vi "WW_GatherSpinParameter.vi"(2 "路径":path) -> (0 "ProgressFinalSpin":T4, 1 "FinalSpinEnd_Index":u32, 3 "RUNStateID":T1, 4 "EXCEL读取":string[][](array[string]), 5 "ProgressInitial":T3, 6 "POWERStateID":T2)   [LabVIEW 2011]
panel:
  # "常用参数：\nPogress_FinalSpin_Index:  用于存储PogressFinalSpinIndex, 用于标定\nFinalSpin_SetpDrain: 用于存储SepDain, 标定\nFinalSpin_StepSpin: 用于活动Spin阶段，进行时间比较\nFinalSpin_StepLoose: 用于活动Loose阶段，标定，而后开始比较"
  # "常用参数：\nPOWER_UPSTGART_Index： 整机正在上电\nPOWER_ON_Idex： 整机处于完全上电状态"
  # "常用参数：\nInitial_StepFirstDrain,(用于计算差价)"
  # "常用参数：\nRUNMODE_READY_Index : 整机准备运行状态\nRUNMODE_RUNNING_Index : 整机处于运行状态"
  # "常用参数：\nFinalSpinEnd_Index: 用于表示数据比对结束"
  # "Useful"
  # "Useful"
  # "Useful"
  # "Useful"
  # "Useful"
  # "Useful"
  # "Useful"
  # "Useful"
  # "Useful"
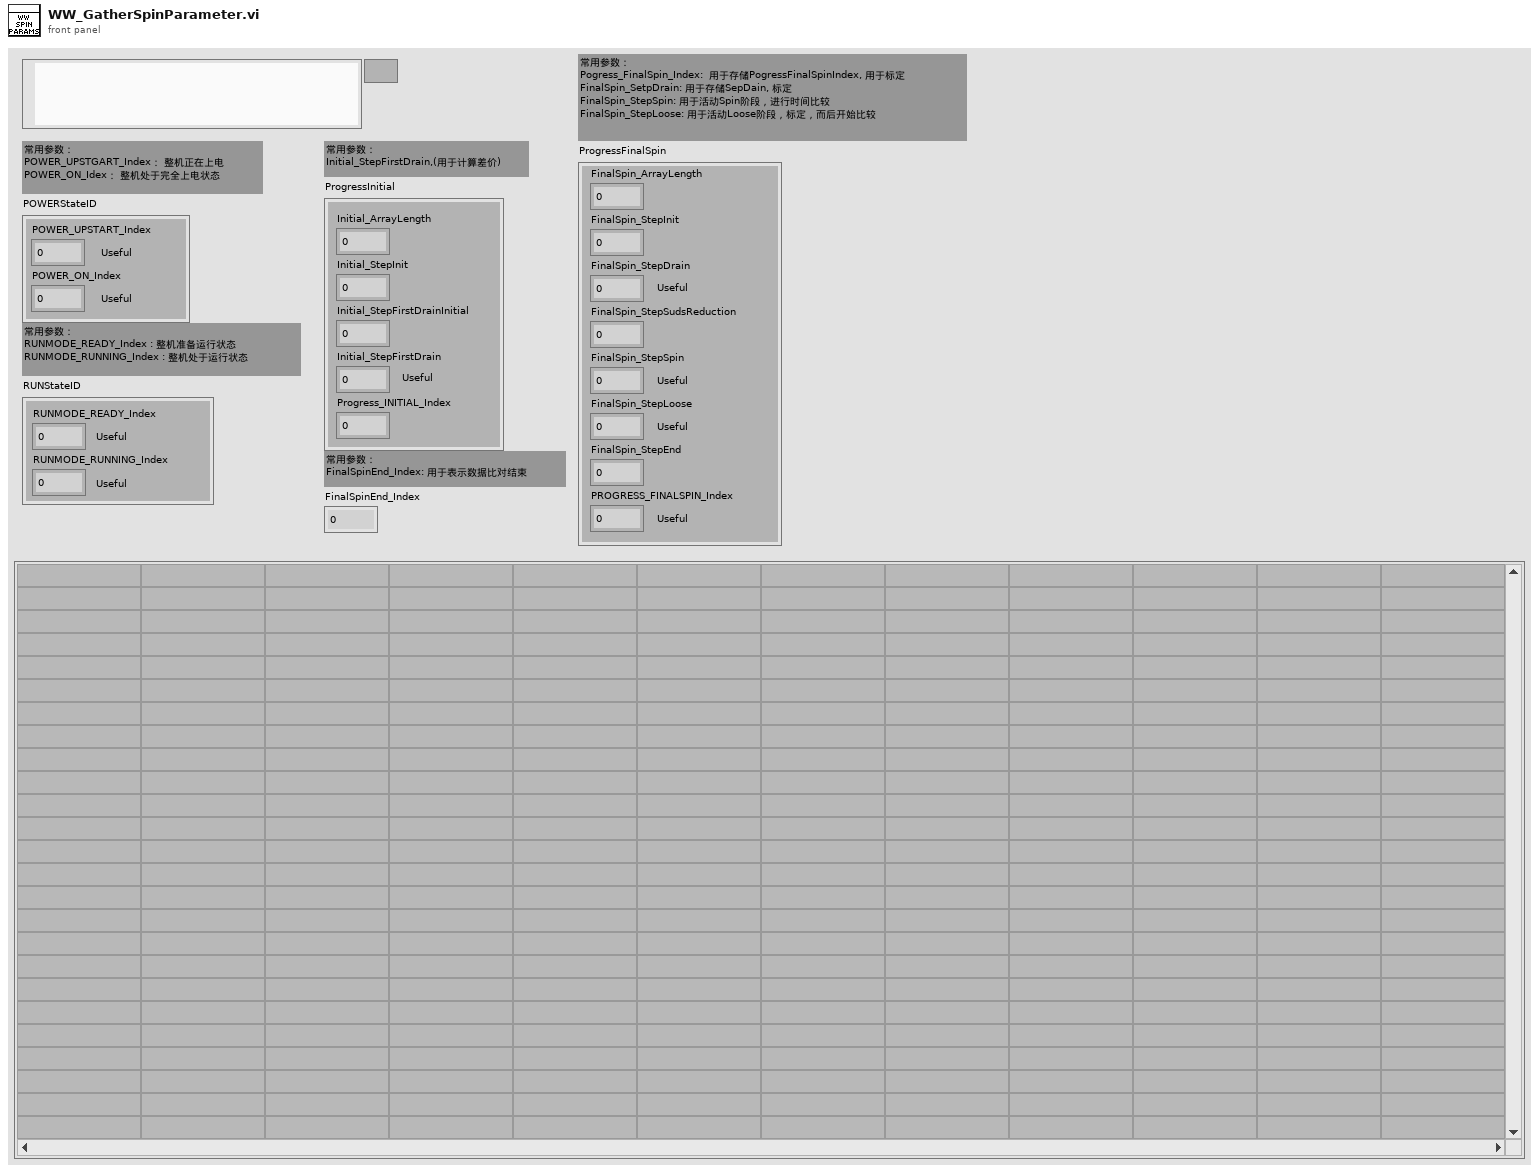
[diagram p1: front panel]
types:
  T1 = cluster{"RUNMODE_READY_Index":u32, "RUNMODE_RUNNING_Index":u32}
  T2 = cluster{"POWER_UPSTART_Index":u32, "POWER_ON_Index":u32}
  T3 = cluster{"Initial_ArrayLength":u32, "Initial_StepInit":u32, "Initial_StepFirstDrainInitial":u32, "Initial_StepFirstDrain":u32, "Progress_INITIAL_Index":u32}
  T4 = cluster{"FinalSpin_ArrayLength":u32, "FinalSpin_StepInit":u32, "FinalSpin_StepDrain":u32, "FinalSpin_StepSudsReduction":u32, "FinalSpin_StepSpin":u32, "FinalSpin_StepLoose":u32, "FinalSpin_StepEnd":u32, "PROGRESS_FINALSPIN_Index":u32}
  T5 = enum16{"RealTime", "WaterLevel", "WaterTemp", "AirTemp", "IPMTemp", "MotorActualRPM", "MotorTargetRPM", "FanActualRPM", "MemsSensorA", "MemsSensorB", "MemsSensorC", "WaterThermistorADC", "TouchSensor", "LeakageSensor", "DCLink", "IsDoorOpen", "IsTimeShort", "Progress", "Step", "TotalRemainTime", "StepRemainTime", "WeightSensingLowData", "WeightSensingResult", "ColdValve", "HotValve", "PreValve", "WaterShotValve", "BleachValve", "DryValve", "SteamValve", "SoftenerValve", "FilterValve", "IsDoorLocked", "SSRCommon", "MainRelay", "ACTUATOR2", "WaterDrainer", "CirculationPump", "WaterHeater", "DryHeater", "SteamHeater", "MotorDriveDirection", "IsDoubleDoorOpen", "IsDoubleDoorLock", "RunStateID", "PowerStateID", "SoundID", "ErrorCode", "OptionData", "MainVersion", "SUBVersion", "InverterVersion"}
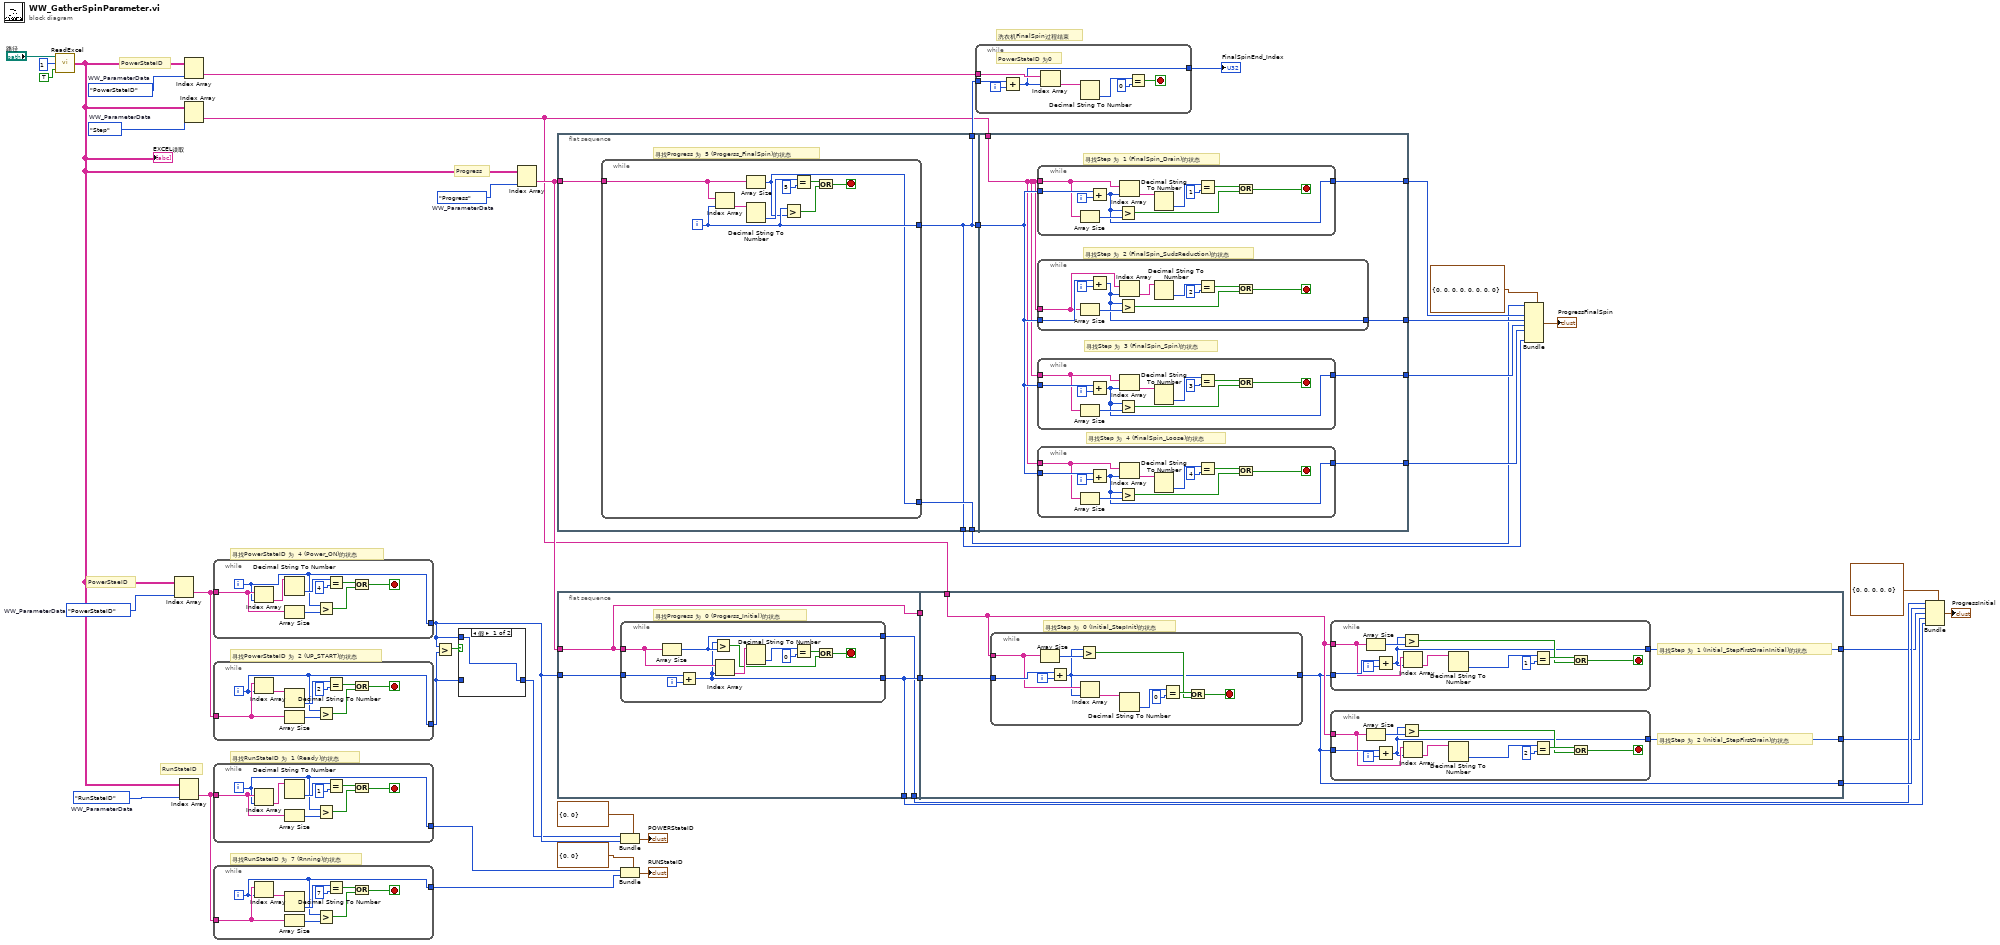
[diagram p0: block diagram]
diagram:
  w6 = T5."RunStateID"  # WW_ParameterData
  w7 = T5."PowerStateID"  # WW_ParameterData
  w9 = T5."Step"  # WW_ParameterData
  w10 = T5."Progress"  # WW_ParameterData
  w11 = T5."PowerStateID"  # WW_ParameterData
  # "PowerStaeID"
  # "洗衣机FinalSpin过程结束"
  # "Progress"
  # "PowerStateID"
  # "RunStateID"
  # "寻找PowerStateID 为  4 (Power_ON)的状态"
  # "寻找PowerStateID 为  2 (UP_START)的状态"
  # "寻找RunStateID 为  1 (Ready)的状态"
  # "寻找RunStateID 为  7 (Rnning)的状态"
  n1 = call "ReadExcel.vi"("读出文本"=TRUE, "导出sheet位号"=i8 1, "路径"="路径") -> ("EXCEL读取"=w12:string[][])
  "EXCEL读取" <- w12
  n2 = Index Array(array=w12, index (col)=w7) -> (element=w40:string[])  [unwired: 1 in]
  n3 = Index Array(array=w12, index (col)=w6) -> (element=w41:string[])  [unwired: 1 in]
  n4 = Index Array(array=w12, index (col)=w11) -> (element=w20:string[])  [unwired: 1 in]
  n5 = Index Array(array=w12, index (col)=w9) -> (element=w8:string[])  [unwired: 1 in]
  n6 = while {
    tunnel: w40 -> [w51]
    tunnel: [w49] -> w2
    i -> [w49]
    stop <- w45 stop-if-true
    n7 = Index Array(array=w51, index=w49) -> (element=w53:string)
    n8 = Decimal String To Number(string=w53) -> (number=w52:i32)  [unwired: 2 in, 1 out]
    n9 = Array Size(array=w51) -> (size(s)=w48:i32)
    n10 = Greater?(x=w49, y=w48) -> (0:w46:bool)
    n11 = Equal?(x=w52, y=4) -> (x = y?=w47:bool)
    n12 = Or(x=w47, y=w46) -> (x .or. y?=w45:bool)
  }
  n13 = while {
    tunnel: w40 -> [w60]
    tunnel: [w58] -> w3
    i -> [w58]
    stop <- w54 stop-if-true
    n14 = Index Array(array=w60, index=w58) -> (element=w62:string)
    n15 = Decimal String To Number(string=w62) -> (number=w61:i32)  [unwired: 2 in, 1 out]
    n16 = Array Size(array=w60) -> (size(s)=w57:i32)
    n17 = Greater?(x=w58, y=w57) -> (0:w55:bool)
    n18 = Equal?(x=w61, y=2) -> (x = y?=w56:bool)
    n19 = Or(x=w56, y=w55) -> (x .or. y?=w54:bool)
  }
  n20 = while {
    tunnel: w41 -> [w69]
    tunnel: [w67] -> w14
    i -> [w67]
    stop <- w63 stop-if-true
    n21 = Index Array(array=w69, index=w67) -> (element=w71:string)
    n22 = Decimal String To Number(string=w71) -> (number=w70:i32)  [unwired: 2 in, 1 out]
    n23 = Array Size(array=w69) -> (size(s)=w66:i32)
    n24 = Greater?(x=w67, y=w66) -> (0:w64:bool)
    n25 = Equal?(x=w70, y=1) -> (x = y?=w65:bool)
    n26 = Or(x=w65, y=w64) -> (x .or. y?=w63:bool)
  }
  n27 = while {
    tunnel: w41 -> [w78]
    tunnel: [w76] -> w13
    i -> [w76]
    stop <- w72 stop-if-true
    n28 = Index Array(array=w78, index=w76) -> (element=w80:string)
    n29 = Decimal String To Number(string=w80) -> (number=w79:i32)  [unwired: 2 in, 1 out]
    n30 = Array Size(array=w78) -> (size(s)=w75:i32)
    n31 = Greater?(x=w76, y=w75) -> (0:w73:bool)
    n32 = Equal?(x=w79, y=7) -> (x = y?=w74:bool)
    n33 = Or(x=w74, y=w73) -> (x .or. y?=w72:bool)
  }
  n34 = Greater?(x=w2, y=w3) -> (0:w5:bool)
  n35 = case shown="假" w5 {
    tunnel: w3 -> [_ w82]
    tunnel: w2 -> [w81 _]
    tunnel: [w81 w82] -> w1
    frame False {
    }
    frame True {
    }
  }
  n36 = Index Array(array=w12, index (col)=w10) -> (element=w28:string[])  [unwired: 1 in]
  n37 = flat-sequence {
    tunnel: w28 -> [w85]
    tunnel: [w83] -> w39
    tunnel: [w83] -> w32
    tunnel: [w84] -> w31
    tunnel: [w83] -> w19
    tunnel: w39 -> [w97]
    tunnel: w8 -> [w96]
    tunnel: [w100] -> w37
    tunnel: [w99] -> w36
    tunnel: [w98] -> w35
    tunnel: [w95] -> w34
    frame #0 {
      # "寻找Progress 为  5 (Progerss_FinalSpin)的状态"
      n38 = while {
        tunnel: w85 -> [w91]
        tunnel: [w87] -> w83
        tunnel: [w86] -> w84
        i -> [w87]
        stop <- w88 stop-if-true
        n39 = Index Array(array=w91, index=w87) -> (element=w94:string)
        n40 = Array Size(array=w91) -> (size(s)=w86:i32)
        n41 = Decimal String To Number(string=w94) -> (number=w93:i32)  [unwired: 2 in, 1 out]
        n42 = Greater?(x=w87, y=w86) -> (0:w89:bool)
        n43 = Equal?(x=w93, y=5) -> (x = y?=w90:bool)
        n44 = Or(x=w90, y=w89) -> (x .or. y?=w88:bool)
      }
    }
    frame #1 {
      # "寻找Step 为  4 (FinalSpin_Loose)的状态"
      # "寻找Step 为  3 (FinalSpin_Spin)的状态"
      # "寻找Step 为  2 (FinalSpin_SudsReduction)的状态"
      # "寻找Step 为  1 (FinalSpin_Drain)的状态"
      n45 = while {
        tunnel: w97 -> [w144]
        tunnel: w96 -> [w134]
        tunnel: [w135] -> w100
        i -> [w143]
        stop <- w136 stop-if-true
        n46 = Array Size(array=w134) -> (size(s)=w139:i32)
        n47 = Add(x=w144, y=w143) -> (x+y=w135:i32)
        n48 = Greater?(x=w135, y=w139) -> (0:w137:bool)
        n49 = Index Array(array=w134, index=w135) -> (element=w142:string)
        n50 = Decimal String To Number(string=w142) -> (number=w141:i32)  [unwired: 2 in, 1 out]
        n51 = Equal?(x=w141, y=1) -> (x = y?=w138:bool)
        n52 = Or(x=w138, y=w137) -> (x .or. y?=w136:bool)
      }
      n53 = while {
        tunnel: w97 -> [w133]
        tunnel: w96 -> [w123]
        tunnel: [w124] -> w99
        i -> [w132]
        stop <- w125 stop-if-true
        n54 = Array Size(array=w123) -> (size(s)=w128:i32)
        n55 = Add(x=w133, y=w132) -> (x+y=w124:i32)
        n56 = Greater?(x=w124, y=w128) -> (0:w126:bool)
        n57 = Index Array(array=w123, index=w124) -> (element=w131:string)
        n58 = Decimal String To Number(string=w131) -> (number=w130:i32)  [unwired: 2 in, 1 out]
        n59 = Equal?(x=w130, y=2) -> (x = y?=w127:bool)
        n60 = Or(x=w127, y=w126) -> (x .or. y?=w125:bool)
      }
      n61 = while {
        tunnel: w97 -> [w122]
        tunnel: w96 -> [w112]
        tunnel: [w113] -> w98
        i -> [w121]
        stop <- w114 stop-if-true
        n62 = Array Size(array=w112) -> (size(s)=w117:i32)
        n63 = Add(x=w122, y=w121) -> (x+y=w113:i32)
        n64 = Greater?(x=w113, y=w117) -> (0:w115:bool)
        n65 = Index Array(array=w112, index=w113) -> (element=w120:string)
        n66 = Decimal String To Number(string=w120) -> (number=w119:i32)  [unwired: 2 in, 1 out]
        n67 = Equal?(x=w119, y=3) -> (x = y?=w116:bool)
        n68 = Or(x=w116, y=w115) -> (x .or. y?=w114:bool)
      }
      n69 = while {
        tunnel: w97 -> [w111]
        tunnel: w96 -> [w101]
        tunnel: [w102] -> w95
        i -> [w110]
        stop <- w103 stop-if-true
        n70 = Array Size(array=w101) -> (size(s)=w106:i32)
        n71 = Add(x=w111, y=w110) -> (x+y=w102:i32)
        n72 = Greater?(x=w102, y=w106) -> (0:w104:bool)
        n73 = Index Array(array=w101, index=w102) -> (element=w109:string)
        n74 = Decimal String To Number(string=w109) -> (number=w108:i32)  [unwired: 2 in, 1 out]
        n75 = Equal?(x=w108, y=4) -> (x = y?=w105:bool)
        n76 = Or(x=w105, y=w104) -> (x .or. y?=w103:bool)
      }
    }
  }
  n77 = flat-sequence {
    tunnel: w28 -> [w147]
    tunnel: [w148] -> w25
    tunnel: [w148] -> w27
    tunnel: [w147] -> w26
    tunnel: [w146] -> w23
    tunnel: w2 -> [w145]
    tunnel: w27 -> [w164]
    tunnel: w26 -> [_]
    tunnel: [w160] -> w24
    tunnel: [w163] -> w22
    tunnel: [w162] -> w21
    tunnel: w8 -> [w161]
    frame #0 {
      # "寻找Progress 为  0 (Progerss_Initial)的状态"
      n78 = while {
        tunnel: w147 -> [w156]
        tunnel: [w150] -> w148
        tunnel: [w152] -> w146
        tunnel: w145 -> [w149]
        i -> [w151]
        stop <- w153 stop-if-true
        n79 = Array Size(array=w156) -> (size(s)=w152:i32)
        n80 = Add(x=w149, y=w151) -> (x+y=w150:i32)
        n81 = Greater?(x=w150, y=w152) -> (0:w154:bool)
        n82 = Index Array(array=w156, index=w150) -> (element=w159:string)
        n83 = Decimal String To Number(string=w159) -> (number=w158:i32)  [unwired: 2 in, 1 out]
        n84 = Equal?(x=w158, y=0) -> (x = y?=w155:bool)
        n85 = Or(x=w155, y=w154) -> (x .or. y?=w153:bool)
      }
    }
    frame #1 {
      # "寻找Step 为  2 (Initial_StepFirstDrain)的状态"
      # "寻找Step 为  1 (Initial_StepFirstDrainInitial)的状态"
      # "寻找Step 为  0 (Initial_StepInit)的状态"
      n86 = while {
        tunnel: w164 -> [w197]
        tunnel: w161 -> [w188]
        tunnel: [w187] -> w160
        i -> [w196]
        stop <- w189 stop-if-true
        n87 = Array Size(array=w188) -> (size(s)=w192:i32)
        n88 = Add(x=w197, y=w196) -> (x+y=w187:i32)
        n89 = Greater?(x=w187, y=w192) -> (0:w190:bool)
        n90 = Index Array(array=w188, index=w187) -> (element=w195:string)
        n91 = Decimal String To Number(string=w195) -> (number=w194:i32)  [unwired: 2 in, 1 out]
        n92 = Equal?(x=w194, y=0) -> (x = y?=w191:bool)
        n93 = Or(x=w191, y=w190) -> (x .or. y?=w189:bool)
      }
      n94 = while {
        tunnel: w160 -> [w186]
        tunnel: w161 -> [w177]
        tunnel: [w176] -> w163
        i -> [w185]
        stop <- w178 stop-if-true
        n95 = Array Size(array=w177) -> (size(s)=w181:i32)
        n96 = Add(x=w186, y=w185) -> (x+y=w176:i32)
        n97 = Greater?(x=w176, y=w181) -> (0:w179:bool)
        n98 = Index Array(array=w177, index=w176) -> (element=w184:string)
        n99 = Decimal String To Number(string=w184) -> (number=w183:i32)  [unwired: 2 in, 1 out]
        n100 = Equal?(x=w183, y=1) -> (x = y?=w180:bool)
        n101 = Or(x=w180, y=w179) -> (x .or. y?=w178:bool)
      }
      n102 = while {
        tunnel: w160 -> [w175]
        tunnel: w161 -> [w166]
        tunnel: [w165] -> w162
        i -> [w174]
        stop <- w167 stop-if-true
        n103 = Array Size(array=w166) -> (size(s)=w170:i32)
        n104 = Add(x=w175, y=w174) -> (x+y=w165:i32)
        n105 = Greater?(x=w165, y=w170) -> (0:w168:bool)
        n106 = Index Array(array=w166, index=w165) -> (element=w173:string)
        n107 = Decimal String To Number(string=w173) -> (number=w172:i32)  [unwired: 2 in, 1 out]
        n108 = Equal?(x=w172, y=2) -> (x = y?=w169:bool)
        n109 = Or(x=w169, y=w168) -> (x .or. y?=w167:bool)
      }
    }
  }
  n110 = Bundle(cluster=cluster{u32, u32} {0, 0}, w1, w2) -> (→"POWERStateID":cluster{u32, u32})
  n111 = Bundle(cluster=cluster{u32, u32} {0, 0}, w14, w13) -> (→"RUNStateID":cluster{u32, u32})
  n112 = while {
    tunnel: w20 -> [w205]
    tunnel: w19 -> [w203]
    tunnel: [w198] -> w18
    i -> [w204]
    stop <- w199 stop-if-true
    # "PowerStateID 为0"
    n113 = Add(x=w203, y=w204) -> (x+y=w198:i32)
    n114 = Index Array(array=w205, index=w198) -> (element=w202:string)
    n115 = Decimal String To Number(string=w202) -> (number=w201:i32)  [unwired: 2 in, 1 out]
    n116 = Equal?(x=w201, y=0) -> (x = y?=w199:bool)
  }
  "FinalSpinEnd_Index" <- w18
  n117 = Bundle(cluster=cluster{u32, u32, u32, u32, u32, u32, u32, u32} {0, 0, 0, 0, 0, 0, 0, 0}, w31, w37, w36, w35, w34, w32) -> (→"ProgressFinalSpin":cluster{u32, u32, u32, u32, u32, u32, u32, u32})  [unwired: 2 in]
  n118 = Bundle(cluster=cluster{u32, u32, u32, u32, u32} {0, 0, 0, 0, 0}, w23, w24, w22, w21, w25) -> (→"ProgressInitial":cluster{u32, u32, u32, u32, u32})
